vi "Save Data.vi"(8 "error in (no error)":errorcluster, 9 "Process Sub Step":string(combo), 10 "Fiber Auto Collimation state data in":refnum<class "Fiber Auto Collimation state data.lvclass">, 11 "Station config in":refnum<class "Station config.lvclass">) -> (0 "error out":errorcluster caption="错误输出", 2 "Fiber Auto Collimation state data out":refnum<class "Fiber Auto Collimation state data.lvclass">, 3 "Station config out":refnum<class "Station config.lvclass">)   [LabVIEW 2018]
uses:
  State data/Fiber Auto Collimation state data.lvclass
  <userlib>/Recipe/Station Config/Station config.lvclass
  C:/Program Files (x86)/National Instruments/LabVIEW 2018/user.lib/Recipe/nLight Recipe/nLight Recipe.lvclass
  State data/String keys.ctl
  State data/Records.ctl
  State data/Fiber Auto Collimation state data.lvclass/Fiber Auto Collimation state data.ctl
  State data/Add Changed data.vi
  <userlib>/Recipe/nLight Recipe/nLight Recipe.lvclass
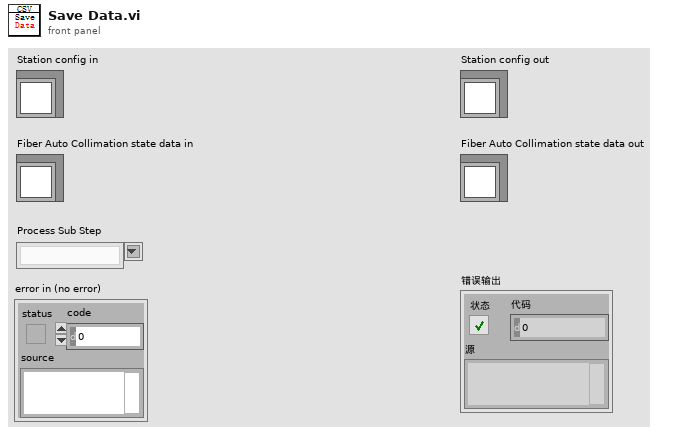
[diagram p1: front panel]
types:
  T1 = typedef "Records.ctl" = cluster{"SN":string, "Test station":string, "MOM Lot":string, "SW Rev":string, "MOM Process":string, "Start time":string, "End time":string, "Knife edge X":dbl, "Peak%Resp":dbl, "Centroid X":dbl, "Knife edge Y":dbl, "Centroid Y":dbl, "Circularity":dbl}
  T2 = typedef "Fiber Auto Collimation state data.lvclass/String keys.ctl" = enum16{"Software version", "Software name", "Collimation Steps Data Path", "Collimation Data Path", "Defect detection Image Path"}
  T3 = typedef "Test Parameters.ctl" = cluster{"Start position":dbl, "Peak Resp_min":dbl, "Circularity_min":dbl, "Beam Size Target":dbl, "Beam Size Percentage ":dbl, "Collimation Steps Data Path":string, "Collimation Data Path":string, "Defect detection Image Path":string, "Save Collimation Steps Data Enable":bool, "Defect detection Enable":bool, "Stop position":dbl}
  T4 = typedef "Fiber Auto Collimation state data.lvclass/Run Time.ctl" = cluster{"Start time":string, "End time":string}
  T5 = typedef "Fiber Auto Collimation state data.lvclass/BV Data.ctl" = cluster{"Centroid X[um]":sgl, "Centroid Y[um]":sgl, "PeakResp.[%]":dbl, "Knife Edge X[mm]":sgl, "Knife Edge Y[mm]":sgl, "Circularity":sgl, "Collimation Result":bool}
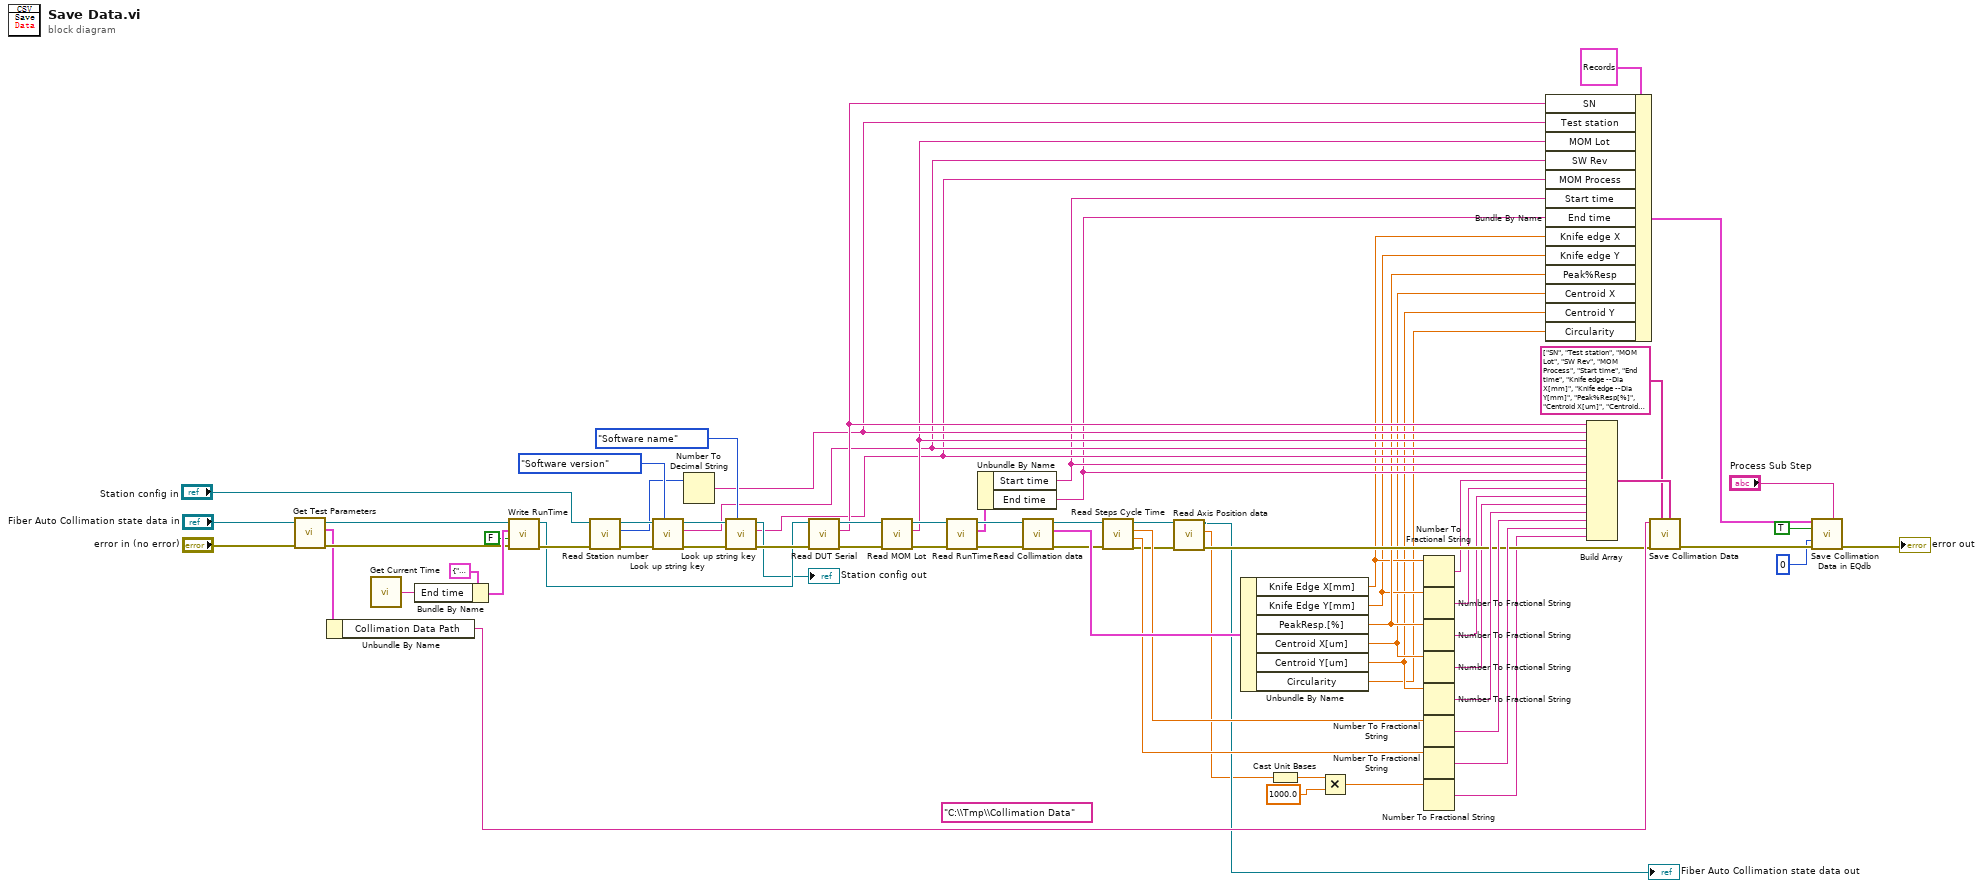
[diagram p0: block diagram]
diagram:
  (unwired) "C:\\Tmp\\Collimation Data" ("路径")
  n1 = call "Get Test Parameters.vi"("error in (no error)"="error in (no error)", "Fiber Auto Collimation state data in"="Fiber Auto Collimation state data in") -> ("error out"=w37:errorcluster, "TestParameters"=w35:T3, "Fiber Auto Collimation state data out"=w38:refnum<class "Fiber Auto Collimation state data.lvclass">)  [unwired: 7 in]
  n2 = Unbundle By Name(w35) -> ("Collimation Data Path"=w34:string)
  n3 = call "Get Current Time.vi"() -> ("日期/时间字符串"=w63:string)  [unwired: 1 in]
  n4 = Bundle By Name(cluster=cluster{"Start time":string, "End time":string} {"Start time"="", "End time"=""} ("Run Time"), "End time"=w63) -> (w61:cluster{"Start time":string, "End time":string})
  n5 = call "Write RunTime.vi"("error in (no error)"=w37, "Start time"=FALSE, "Run Time"=w61, "Fiber Auto Collimation state data in"=w38) -> ("error out"=w60:errorcluster, "Fiber Auto Collimation state data out"=w48:refnum<class "Fiber Auto Collimation state data.lvclass">)  [unwired: 6 in]
  n6 = call-dynamic "Read Station number.vi"("error in (no error)"=w60, "Station config in"="Station config in") -> ("error out"=w71:errorcluster, "Station number"=w55:i32, "Station config out"=w70:refnum<class "Station config.lvclass">)  [unwired: 7 in]
  n7 = call <userlib>:"Look up string key.vi"("Key [string/enum]"=String_keys."Software version" ("Station config string keys"), "error in (no error)"=w71, "nLight Recipe in"=w70) -> ("error out"=w67:errorcluster, "String Key Value"=w20:string, "nLight Recipe out"=w65:refnum<class "Station config.lvclass">)  [unwired: 5 in, 1 out]
  n8 = Number To Decimal String(number=w55) -> (decimal integer string=w22:string)  [unwired: 1 in]
  n9 = call <userlib>:"Look up string key.vi"("Key [string/enum]"=String_keys."Software name" ("Station config string keys"), "error in (no error)"=w67, "nLight Recipe in"=w65) -> ("error out"=w66:errorcluster, "String Key Value"=w19:string, "nLight Recipe out"=→"Station config out":refnum<class "Station config.lvclass">)  [unwired: 5 in, 1 out]
  n10 = call "Read DUT Serial.vi"("error in (no error)"=w66, "Fiber Auto Collimation state data in"=w48) -> ("error out"=w69:errorcluster, "DUT Serial"=w23:string, "Fiber Auto Collimation state data out"=w62:refnum<class "Fiber Auto Collimation state data.lvclass">)  [unwired: 7 in]
  n11 = call "Read MOM Lot.vi"("error in (no error)"=w69, "Fiber Auto Collimation state data in"=w62) -> ("error out"=w58:errorcluster, "MOM Lot"=w21:string, "Fiber Auto Collimation state data out"=w59:refnum<class "Fiber Auto Collimation state data.lvclass">)  [unwired: 7 in]
  n12 = call "Read RunTime.vi"("error in (no error)"=w58, "Fiber Auto Collimation state data in"=w59) -> ("error out"=w56:errorcluster, "Run Time"=w54:T4, "Fiber Auto Collimation state data out"=w57:refnum<class "Fiber Auto Collimation state data.lvclass">)  [unwired: 7 in]
  n13 = Unbundle By Name(w54) -> ("Start time"=w18:string, "End time"=w17:string)
  n14 = call "Read Collimation data.vi"("error in (no error)"=w56, "Fiber Auto Collimation state data in"=w57) -> ("error out"=w45:errorcluster, "BV Data"=w52:T5, "Fiber Auto Collimation state data out"=w44:refnum<class "Fiber Auto Collimation state data.lvclass">)  [unwired: 7 in]
  n15 = call "Read Steps Cycle Time.vi"("error in (no error)"=w45, "Fiber Auto Collimation state data in"=w44) -> ("error out"=w33:errorcluster, "Defect detection Time"=w42:dbl, "Collimation Time"=w43:dbl, "Fiber Auto Collimation state data out"=w31:refnum<class "Fiber Auto Collimation state data.lvclass">)  [unwired: 6 in]
  n16 = call "Read Axis Position data.vi"("error in (no error)"=w33, "Fiber Auto Collimation state data in"=w31) -> ("error out"=w32:errorcluster, "Current position"=w29:dbl[unit], "Fiber Auto Collimation state data out"=→"Fiber Auto Collimation state data out":refnum<class "Fiber Auto Collimation state data.lvclass">)  [unwired: 7 in]
  n17 = Unbundle By Name(w52) -> ("Knife Edge X[mm]"=w11:sgl, "Knife Edge Y[mm]"=w10:sgl, "PeakResp.[%]"=w12:dbl, "Centroid X[um]"=w9:sgl, "Centroid Y[um]"=w8:sgl, "Circularity"=w7:sgl)
  n18 = Cast Unit Bases(0:w29) -> (2:w28:dbl)  [unwired: 1 in]
  n19 = Multiply(x=w28, y=1000.0) -> (x*y=w26:dbl)
  n20 = Number To Fractional String(number=w11) -> (F-format string=w16:string)  [unwired: 3 in]
  n21 = Number To Fractional String(number=w10) -> (F-format string=w15:string)  [unwired: 3 in]
  n22 = Number To Fractional String(number=w12) -> (F-format string=w14:string)  [unwired: 3 in]
  n23 = Number To Fractional String(number=w9) -> (F-format string=w13:string)  [unwired: 3 in]
  n24 = Number To Fractional String(number=w8) -> (F-format string=w51:string)  [unwired: 3 in]
  n25 = Number To Fractional String(number=w43) -> (F-format string=w41:string)  [unwired: 3 in]
  n26 = Number To Fractional String(number=w42) -> (F-format string=w40:string)  [unwired: 3 in]
  n27 = Number To Fractional String(number=w26) -> (F-format string=w25:string)  [unwired: 3 in]
  n28 = Bundle By Name(cluster=T1 {"SN"="", "Test station"="", "MOM Lot"="", "SW Rev"="", "MOM Process"="", "Start time"="", "End time"="", "Knife edge X"=0.0, "Peak%Resp"=0.0, "Centroid X"=0.0, "Knife edge Y"=0.0, "Centroid Y"=0.0, "Circularity"=0.0}, "SN"=w23, "Test station"=w22, "MOM Lot"=w21, "SW Rev"=w20, "MOM Process"=w19, "Start time"=w18, "End time"=w17, "Knife edge X"=w11, "Knife edge Y"=w10, "Peak%Resp"=w12, "Centroid X"=w9, "Centroid Y"=w8, "Circularity"=w7) -> (w4:T1)
  n29 = Build Array(w23, w22, w21, w20, w19, w18, w17, w16, w15, w14, w13, w51, w41, w40, w25) -> (w53:string[])
  n30 = call "Save Collimation Data.vi"("Data"=w53, "Item"=string[] ["SN", "Test station", "MOM Lot", "SW Rev", "MOM Process", "Start time", "End time", "Knife edge --Dia X[mm]", "Knife edge --Dia Y[mm]", "Peak%Resp[%]", "Centroid X[um]", "Centroid Y[um]", "Collimation Time[s]", "Defect detection Time[s]", "Collimation Position[mm]"], "Error In"=w32, "路径"=w34) -> ("error out"=w5:errorcluster)  [unwired: 7 in]
  n31 = call "Save Collimation Data in EQdb.vi"("Records"=w4, "Process Sub Step"="Process Sub Step", "Process to LEQdb"=TRUE, "TestNumber"=0, "error in (no error)"=w5) -> ("error out"=→"error out":errorcluster)  [unwired: 8 in, 2 out]
